vi "read timing source name.vi"(8 "error in":errorcluster, 11 "module in":refnum<class "TBM module execution interface.lvclass">) -> (0 "error out":errorcluster, 2 "timing source":refnum<class "TBM timing source.lvclass">, 3 "module out":refnum<class "TBM module execution interface.lvclass">)   [LabVIEW 2013, in "TBM module execution interface.lvclass"]
doc: "Retrieves a timing source name from the module, if configured. An empty string is defined as meaning that no timing source exists."
uses:
  TBM module execution interface.lvclass
  <vilib>/NI/Module Timing Source/timing source/TBM timing source.lvclass
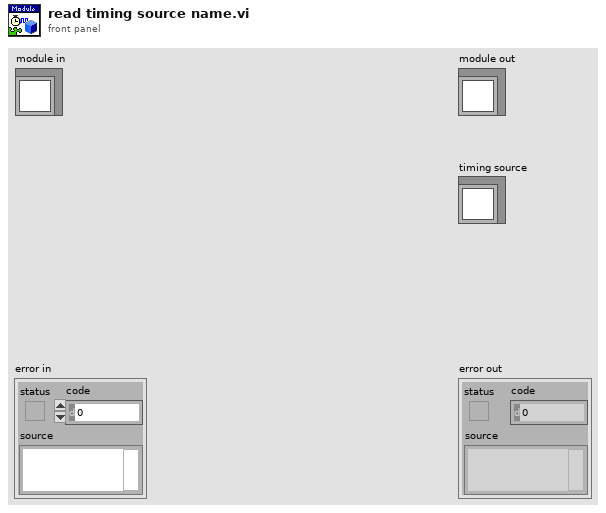
[diagram p1: front panel]
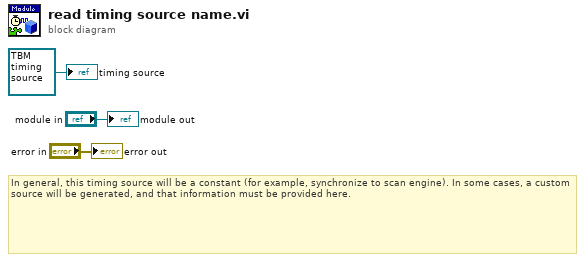
[diagram p0: block diagram]
diagram:
  # "In general, this timing source will be a constant (for example, synchronize to scan engine). In some cases, a custom source will be generated, and that information must be provided here."
  "error out" <- "error in"
  "module out" <- "module in"
  "timing source" <- refnum<class "TBM timing source.lvclass"> refnum ("TBM Timing Source in")
